vi "Create Command Frame FCS.vi"(0 "USID":u8=2, 1 "Address":u8=24 format="%.0x", 2 "Command_WriteF":u8=4 format="%.0x", 3 "Num_of_FCS_Bits":u8=5, 4 "Polynomial_Mask":u8=37 format="%.0x", 5 "error in (no error)":errorcluster, 6 "OVS":u8=16, 7 "sample rate":dbl=1000.0 format="%#_6p") -> (14 "Digital Waveform Graph_Out":digitalwaveform(graph), 19 "error out":errorcluster)   [LabVIEW 2013]
panel:
  out "Final_Command_Frame":bool[](array[boolean])
  out "All_Decoding_Steps":bool[][](array[boolean])
  out "FCS_Value":i32
  out "Final_CMD_FCS":bool[](array[boolean])
  out "Command_FCS":bool[](array[boolean])
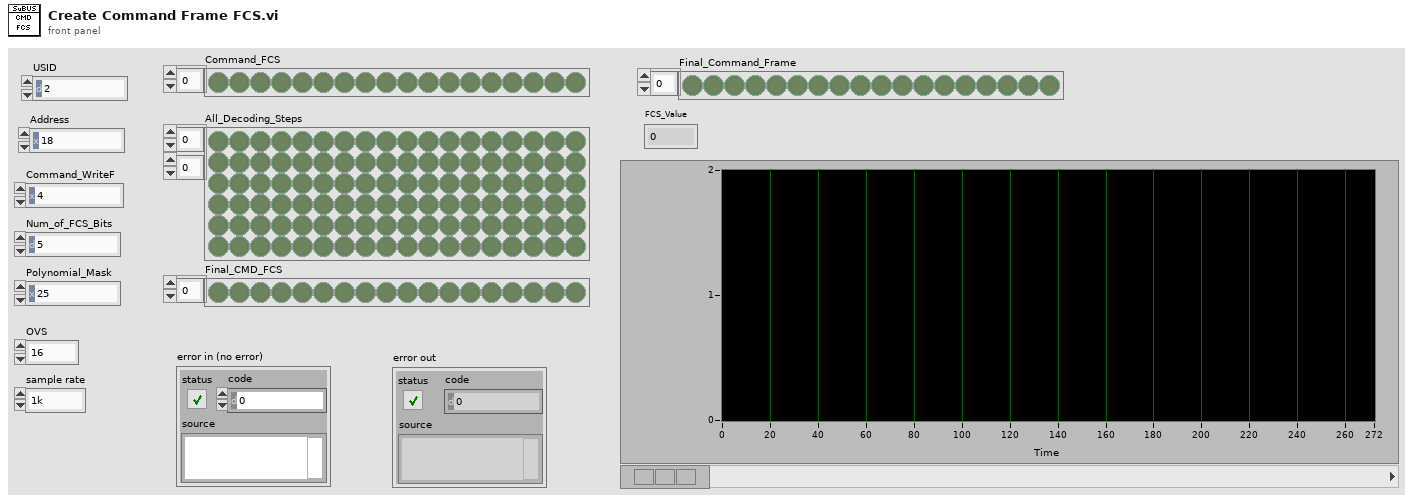
[diagram p1: front panel]
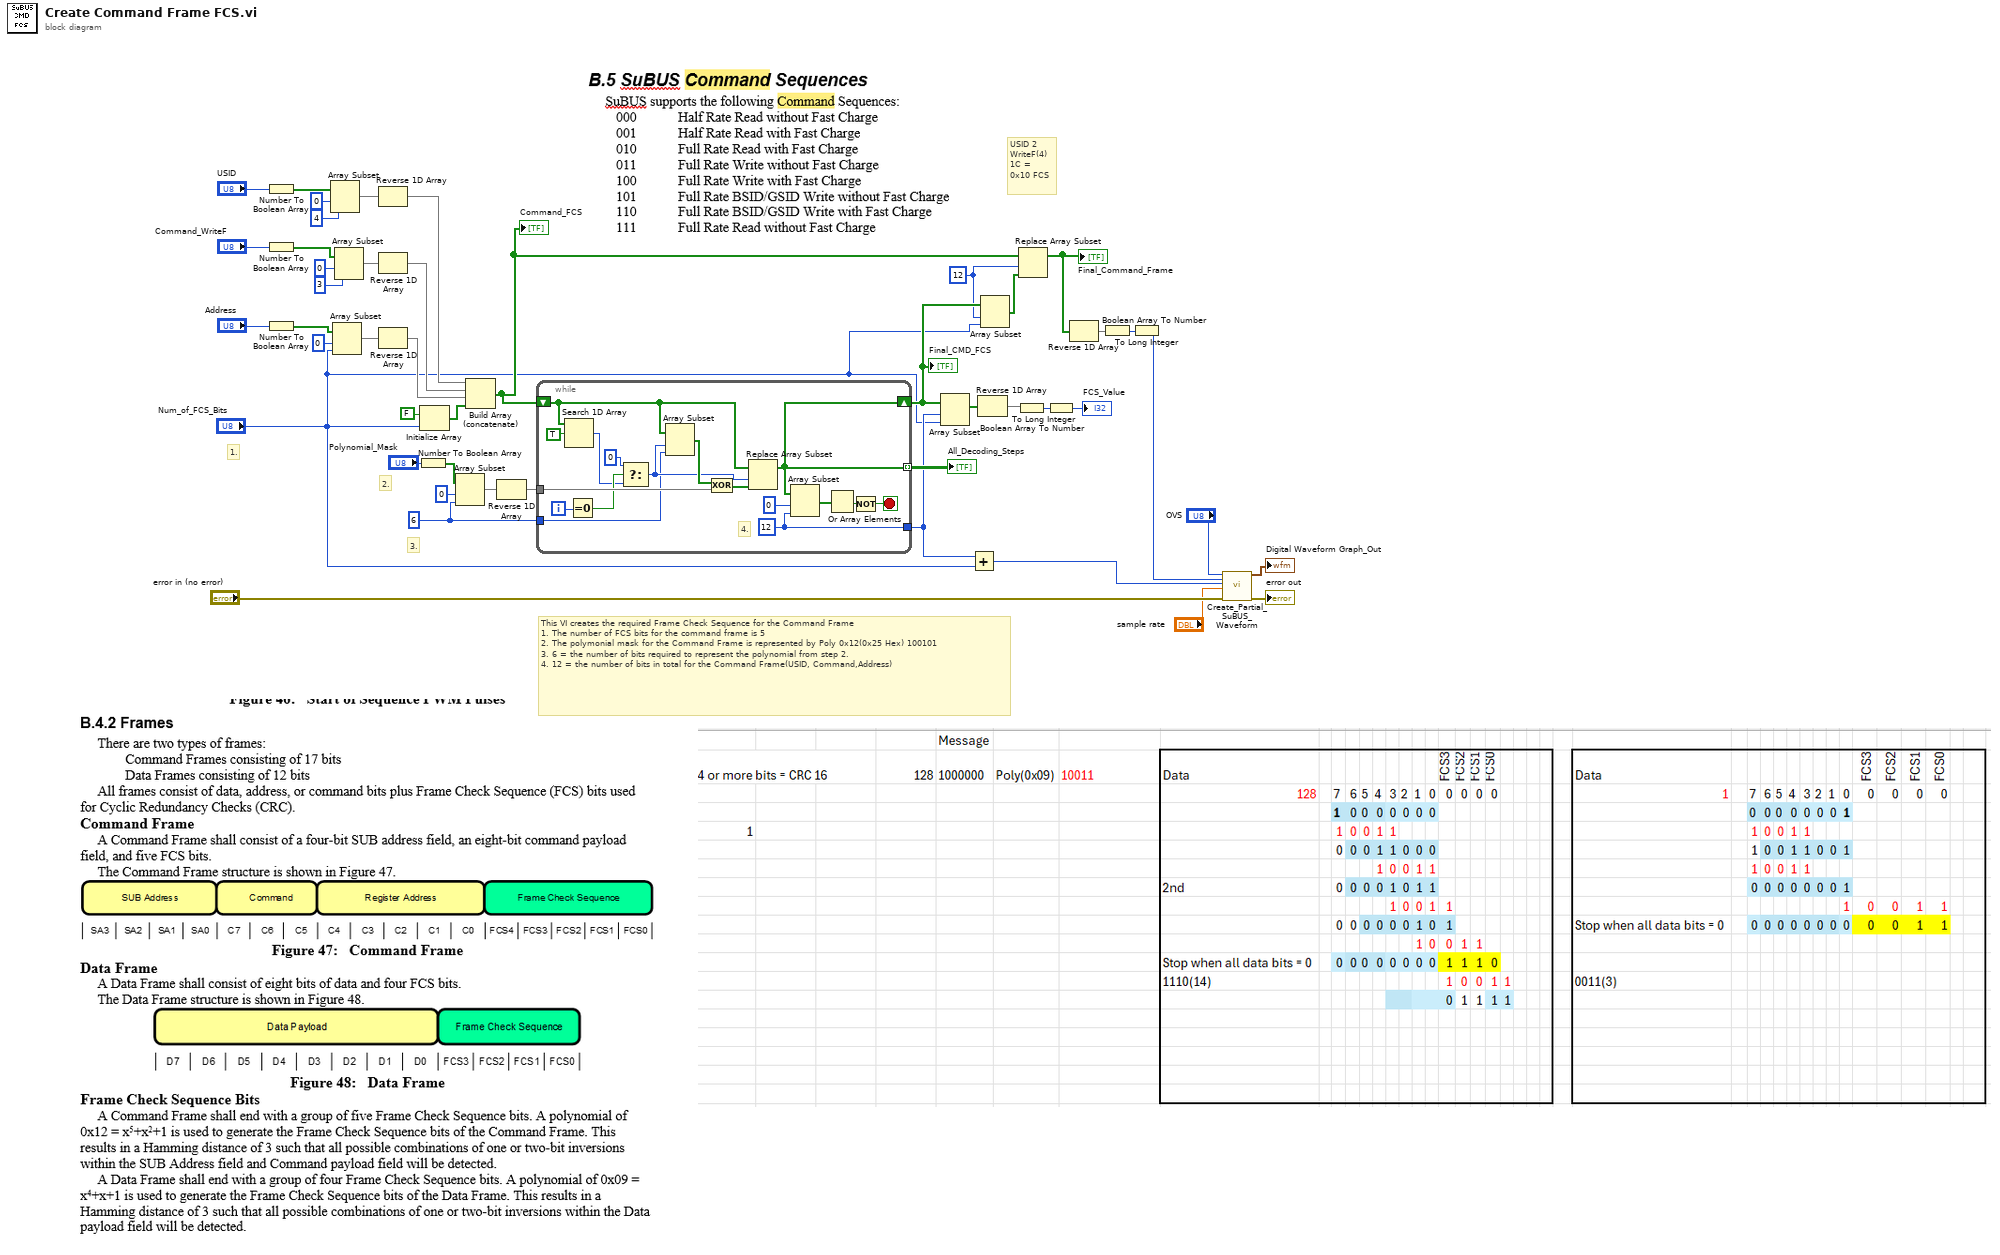
[diagram p0: block diagram]
diagram:
  w1 = 12 ("index")
  w37 = 6 ("length")
  # "This VI creates the required Frame Check Sequence for the Command Frame\n1. The number of FCS bits for the command frame is 5 \n2. The polymonial mask for the Command Frame is represented by Poly 0x12(0x25 Hex) 100101\n3. 6 = the number of bits required to represent the polynomial from step 2.\n4. 12 = the number of bits in total for the Command Frame(USID, Command,Address)"
  # "3."
  # "2."
  # "1."
  # "USID 2\nWriteF(4)\n1C = \n0x10 FCS"
  n1 = Number To Boolean Array(number="USID") -> (Boolean array=w29:bool[])
  n2 = Number To Boolean Array(number="Command_WriteF") -> (Boolean array=w30:bool[])
  n3 = Number To Boolean Array(number="Address") -> (Boolean array=w24:bool[])
  n4 = Array Subset(array=w29, index=0, length=4) -> (w28:bool[])
  n5 = Array Subset(array=w24, index=0, length="Num_of_FCS_Bits") -> (w23:bool[])
  n6 = Array Subset(array=w30, index=0, length=3) -> (w26:bool[])
  n7 = Reverse 1D Array(array=w28) -> (reversed array=w27:bool[])
  n8 = Reverse 1D Array(array=w26) -> (reversed array=w25:bool[])
  n9 = Reverse 1D Array(array=w23) -> (reversed array=w22:bool[])
  n10 = Number To Boolean Array(number="Polynomial_Mask") -> (Boolean array=w46:bool[])
  n11 = Initialize Array(FALSE ("element"), "Num_of_FCS_Bits") -> (w43:bool[])
  n12 = Array Subset(array=w46, index=0, length=w37) -> (w45:bool[])
  n13 = Build Array (concatenate)(w27, w25, w22, w43) -> (w7:bool[])
  "Command_FCS" <- w7
  n14 = Reverse 1D Array(array=w45) -> (reversed array=w42:bool[])
  n15 = while {
    shift-right: [w49] -> w6
    shift-left: w7 -> [w56]
    tunnel: w42 -> [w63]
    tunnel: [w49] -> w40 mode=indexing
    tunnel: w37 -> [w48]
    tunnel: [w47] -> w11
    i -> [w54]
    stop <- w57 stop-if-true
    w47 = 12 ("length")
    # "4."
    n16 = Search 1D Array(1D array=w56, element=TRUE) -> (index of element=w52:i32)  [unwired: 1 in]
    n17 = Equal To 0?(x=w54) -> (x = 0?=w53:bool)
    n18 = Select(t=0, s=w53, f=w52) -> (s? t:f=w51:i32)
    n19 = Array Subset(array=w56, index=w51, length=w48) -> (w62:bool[])
    n20 = Exclusive Or(1:w63, 2:w62) -> (0:w55:bool[])
    n21 = Replace Array Subset(array=w56, new element=w55, index=w51) -> (w49:bool[])
    n22 = Array Subset(array=w49, index=0, length=w47) -> (w60:bool[])
    n23 = Or Array Elements(Boolean array=w60) -> (logical OR=w59:bool)
    n24 = Not(x=w59) -> (.not. x?=w57:bool)
  }
  "Final_CMD_FCS" <- w6
  "All_Decoding_Steps" <- w40
  n25 = Array Subset(array=w6, index=w11, length="Num_of_FCS_Bits") -> (w41:bool[])
  n26 = Add(x=w11, y="Num_of_FCS_Bits") -> (x+y=w8:i32)
  n27 = Reverse 1D Array(array=w41) -> (reversed array=w14:bool[])
  n28 = Array Subset(array=w6, index=w1, length="Num_of_FCS_Bits") -> (w5:bool[])
  n29 = Boolean Array To Number(Boolean array=w14) -> (number=w21:u32)
  n30 = Replace Array Subset(array=w7, new element=w5, index=w1) -> (w4:bool[])
  "Final_Command_Frame" <- w4
  n31 = To Long Integer(number=w21) -> (32bit integer=→"FCS_Value":i32)
  n32 = Reverse 1D Array(array=w4) -> (reversed array=w3:bool[])
  n33 = Boolean Array To Number(Boolean array=w3) -> (number=w13:u32)
  n34 = To Long Integer(number=w13) -> (32bit integer=w12:i32)
  n35 = call "Create_Partial_SuBUS_Waveform.vi"("OVS"="OVS", "Value"=w12, "Bit_length"=w8, "sample rate"="sample rate", "error in (no error)"="error in (no error)") -> ("Digital Waveform Graph_Out"=→"Digital Waveform Graph_Out":digitalwaveform, "error out"=→"error out":errorcluster)  [unwired: 13 in]
